vi "update camera op mode error.vi"(8 "error in (no error)":errorcluster, 11 "Channel in":refnum<class "SPARC4_Channel.lvclass">) -> (0 "error out":errorcluster, 3 "Channel out":refnum<class "SPARC4_Channel.lvclass">)   [LabVIEW 2018, in "SPARC4_Channel.lvclass"]
doc: "Verify if there is an error in the error array of the camera class\n\nThis function will return true if there is any error or warning in the error array of the camera with a code different of 20002 or 0."
uses:
  SPARC4_Channel.lvclass
  <vilib>/ErrorRing/Error Ring.xnode
  <vilib>/Utility/error.llb/Error Cluster From Error Code.vi
  Sim_CCD/Sim_CCD.lvclass
  Sim_Ixon_Ultra/Sim_Ixon_Ultra.lvclass
  C:/Users/Denis/Desktop/S4ACS/S4ACS/Sim_CCD/Sim_CCD.lvclass
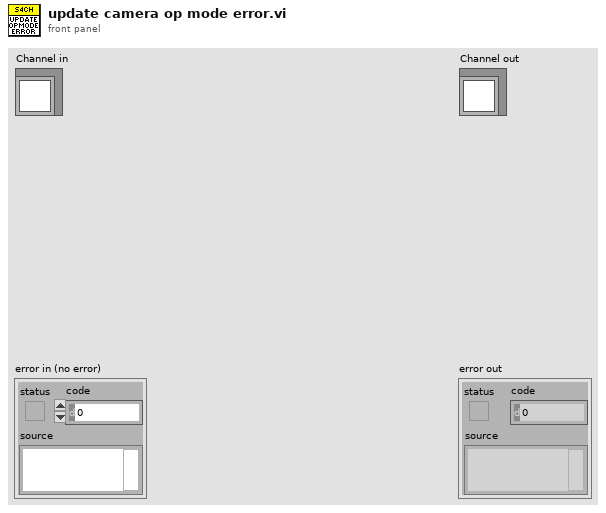
[diagram p1: front panel]
types:
  T1 = cluster{"EXPTIME":errorcluster, "#FRAMES":errorcluster}
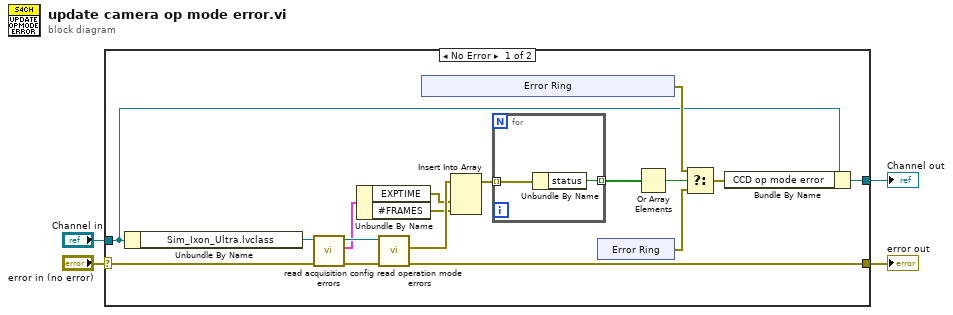
[diagram p0: block diagram]
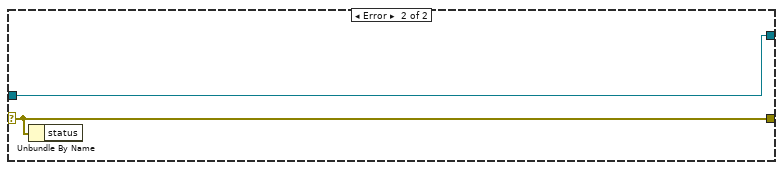
[diagram p2: hidden frame]
diagram:
  n1 = case shown="No Error" "error in (no error)" {
    selector: "error in (no error)" -> [w10 w30]
    tunnel: [w16 w30] -> w3
    tunnel: [w21 w31] -> w1
    tunnel: "Channel in" -> [w17 w31]
    frame No Error {
      n2 = Unbundle By Name(w17) -> ("Sim_Ixon_Ultra.lvclass"=w13:refnum<class "Sim_Ixon_Ultra.lvclass">)
      n3 = call "read acquisition config errors.vi"("error in (no error)"=w10, "Simulated Camera in"=w13) -> ("error out"=w11:errorcluster, "acq config errors"=w8:T1, "Simulated Camera out"=w12:refnum<class "Sim_Ixon_Ultra.lvclass">)  [unwired: 7 in]
      n4 = Unbundle By Name(w8) -> ("EXPTIME"=w6:errorcluster, "#FRAMES"=w5:errorcluster)
      n5 = call "read operation mode errors.vi"("error in (no error)"=w11, "Simulated_CCD_Camera in"=w12) -> ("error out"=w16:errorcluster, "WRITE SETUP errors"=w7:errorcluster[])  [unwired: 7 in, 1 out]
      n6 = xnode "Error Ring"() -> ("error out"=w20:errorcluster)
      n7 = Insert Into Array(array=w7, new element #1=w6, new element #2=w5) -> (w9:errorcluster[])  [unwired: 1 in]
      n8 = for {
        tunnel: w9 -> [w23] mode=indexing
        tunnel: [w22] -> w14 mode=indexing
        n9 = Unbundle By Name(w23) -> ("status"=w22:bool)
      }
      n10 = xnode "Error Ring"() -> ("error out"=w18:errorcluster)
      n11 = Or Array Elements(Boolean array=w14) -> (logical OR=w15:bool)
      n12 = Select(t=w20, s=w15, f=w18) -> (s? t:f=w19:errorcluster)
      n13 = Bundle By Name(cluster=w17, "CCD op mode error"=w19) -> (w21:refnum<class "SPARC4_Channel.lvclass">)
    }
    frame Error {
      n14 = Unbundle By Name(w30) -> ()  [unwired: 1 out]
    }
  }
  "error out" <- w3
  "Channel out" <- w1
